vi "Vision.vi"   [LabVIEW 2016]
uses:
  Robot Global Data.vi
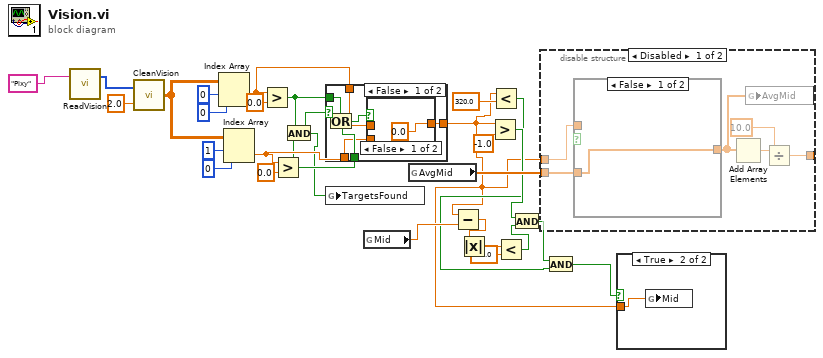
[diagram p0: block diagram]
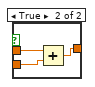
[diagram p2: hidden frame]
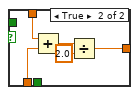
[diagram p3: hidden frame]
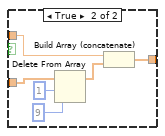
[diagram p5: hidden frame]
diagram:
  n1 = call "ReadVision.vi"("Name"="Pixy") -> ("Target Data"=w27:u16[])  [unwired: 2 in]
  n2 = call "CleanVision.vi"("Targets"=2.0, "Input"=w27) -> ("Output"=w23:dbl[][])
  n3 = Index Array(array=w23, index (row)=0, index (col)=0 ("disabled index (col)")) -> (element=w5:dbl)
  n4 = Index Array(array=w23, index (row)=1, index (col)=0 ("disabled index (col)")) -> (element=w4:dbl)
  n5 = Greater?(x=w5, y=0.0) -> (0:w3:bool)
  n6 = Greater?(x=w4, y=0.0) -> (0:w2:bool)
  n7 = And(x=w3, y=w2) -> (x .and. y?=w1:bool)
  n8 = case shown="False" w1 {
    tunnel: [w30 w41] -> w8
    tunnel: w5 -> [w31 w40]
    tunnel: w4 -> [w32 w39]
    tunnel: w3 -> [w34 _]
    tunnel: w2 -> [w33 _]
    frame False {
      n9 = Or(x=w34, y=w33) -> (x .or. y?=w29:bool)
      n10 = case shown="False" w29 {
        tunnel: w32 -> [_ w38]
        tunnel: w31 -> [_ w37]
        tunnel: [0.0 w36] -> w30
        frame False {
        }
        frame True {
          n11 = Add(x=w37, y=w38) -> (x+y=w36:dbl)
        }
      }
    }
    frame True {
      n12 = Add(x=w40, y=w39) -> (x+y=w43:dbl)
      n13 = Divide(x=w43, y=2.0) -> (x/y=w41:dbl)
    }
  }
  n14 = global write "Robot Global Data.vi" "TargetsFound"(w1) -> ()
  n15 = global read "Robot Global Data.vi" "Mid"() -> (w16:dbl)
  n16 = global read "Robot Global Data.vi" "AvgMid"() -> (w18:dbl[])
  n17 = Subtract(x=w8, y=w16) -> (x-y=w15:dbl)
  n18 = Absolute Value(x=w15) -> (abs(x)=w14:dbl)
  n19 = Greater?(x=w8, y=-1.0) -> (0:w17:bool)
  n20 = Less?(x=w8, y=320.0) -> (x < y?=w10:bool)
  n21 = Less?(x=w14, y=300.0) -> (x < y?=w12:bool)
  n22 = And(x=w17, y=w12) -> (x .and. y?=w11:bool)
  n23 = disable-structure shown="Disabled" {
    disable-tunnel: w18 -> [w49 _]
    disable-tunnel: [w45 _] -> _
    disable-tunnel: w8 -> [w44 _]
    frame Disabled {
      n24 = case shown="False" w50 {
        tunnel: w49 -> [w51 w57]
        tunnel: w44 -> [_ w53]
        tunnel: [w51 w52] -> w46
        frame False {
        }
        frame True {
          n25 = Delete From Array(array=w57, length=1, index=9) -> (array with subset deleted=w54:dbl[])  [unwired: 1 out]
          n26 = Build Array (concatenate)(w53, w54) -> (w52:dbl[])
        }
      }
      n27 = Add Array Elements(numeric array=w46) -> (sum=w48:dbl)
      n28 = global write "Robot Global Data.vi" "AvgMid"(w46) -> ()
      n29 = Divide(x=w48, y=10.0) -> (x/y=w45:dbl)
    }
    frame Enabled {
    }
  }
  n30 = And(x=w11, y=w10) -> (x .and. y?=w9:bool)
  n31 = case shown="True" w9 {
    tunnel: w8 -> [_ w58]
    frame False {
    }
    frame True {
      n32 = global write "Robot Global Data.vi" "Mid"(w58) -> ()
    }
  }
